vi "Parse And Send VISA Command String.vi"(8 "error in":errorcluster, 10 "command":string, 11 "VISA in":refnum<visa-resource-name>) -> (0 "error out":errorcluster, 2 "fetch data":T1[](array[typedef]), 3 "VISA out":refnum<visa-resource-name>)   [LabVIEW 2020]
uses:
  Raw VISA Read Data.ctl
  <vilib>/Instr/_visa.llb/VISA GPIB Control REN Mode.ctl
  <vilib>/Instr/_visa.llb/VISA Flush IO Buffer Mask.ctl
  Raw VISA Read Data.vi
  <vilib>/regexp/Match Regular Expression.xnode
  varilib/varilib.lvlib
panel:
  out "result string":string
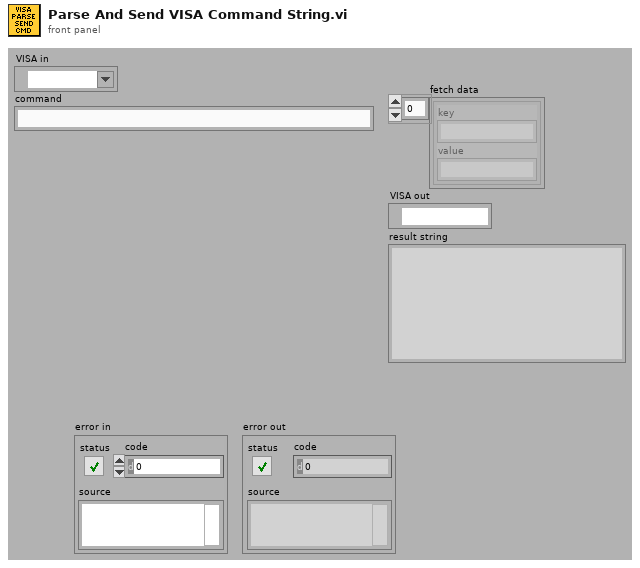
[diagram p1: front panel]
types:
  T1 = typedef "Raw VISA Read Data.ctl" = cluster{"key":string, "value":string}
  T2 = cluster{"submatch 2":string, "trimmed string":string}[]
  T3 = typedef "Raw VISA Read Data.vi" = cluster{"key":string, "value":string}
  T4 = typedef "VISA GPIB Control REN Mode.ctl" = u16
  T5 = typedef "VISA Flush IO Buffer Mask.ctl" = u16
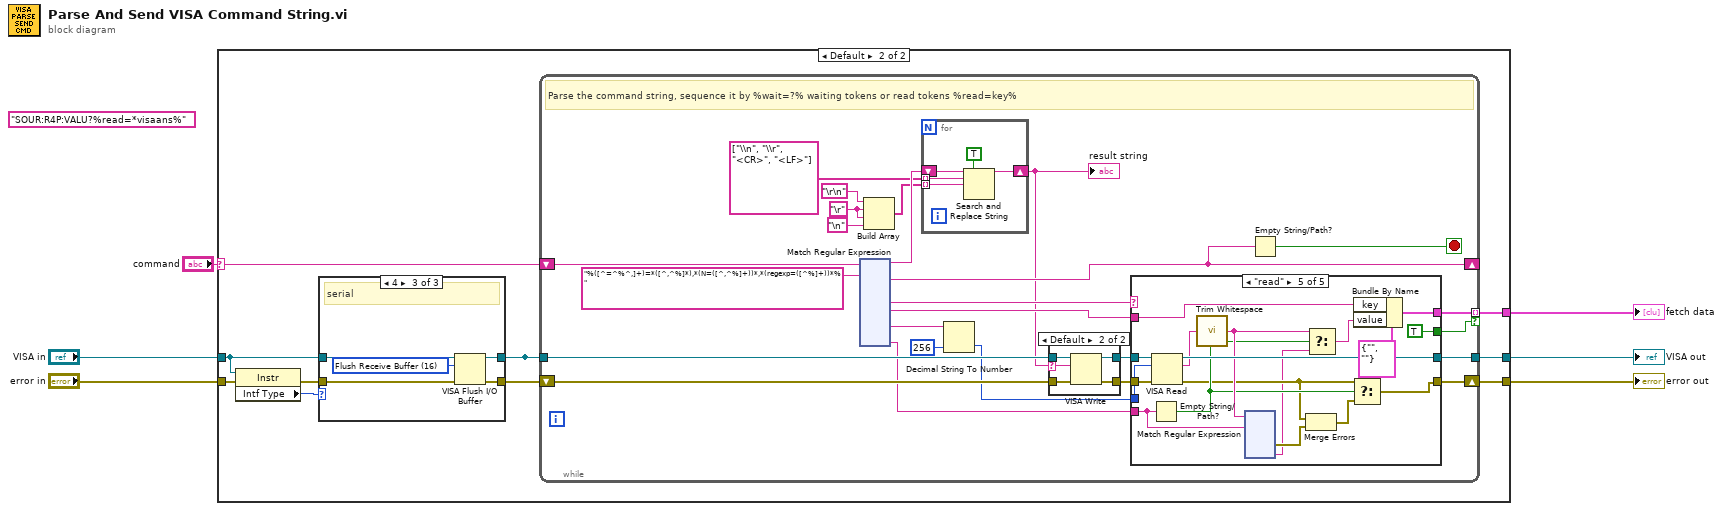
[diagram p0: block diagram]
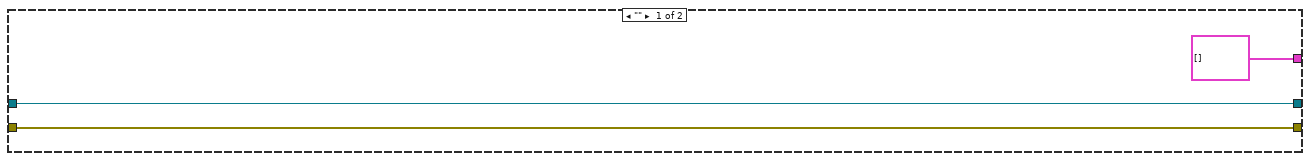
[diagram p2: hidden frame]
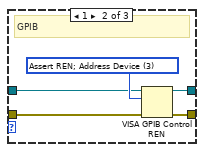
[diagram p4: hidden frame]
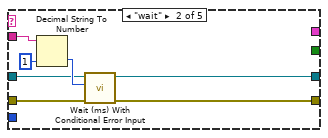
[diagram p7: hidden frame]
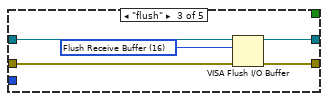
[diagram p8: hidden frame]
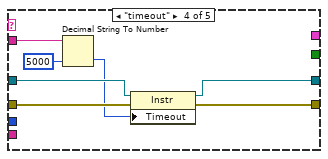
[diagram p9: hidden frame]
diagram:
  (unwired) "SOUR:R4P:VALU?%read=*visaans%"
  n1 = case shown="Default" "command" {
    selector: "command" -> [_ w17]
    tunnel: "error in" -> [w9 w12]
    tunnel: [w9 w18] -> w5
    tunnel: "VISA in" -> [w8 w13]
    tunnel: [w8 w15] -> w3
    tunnel: [T2 [] ("Array") w14] -> w4
    frame "" {
    }
    frame Default {
      n2 = property class="Instr"(reference=w13, error in=w12) -> (error out=w11:errorcluster, "Intf Type"=w10:u16)  [unwired: 1 out]
      n3 = case shown="4" w10 {
        tunnel: [w20 w25 w29] -> w16
        tunnel: [w19 w23 w28] -> w15
        tunnel: w13 -> [w19 w22 w27]
        tunnel: w11 -> [w20 w21 w30]
        frame 0, Default {
        }
        frame 1 {
          w24 = T4 3 items=["Deassert REN", "Assert REN", "Go To Local; Deassert REN ", "Assert REN; Address Device", "Local Lockout (Addressed Devices)", "Local Lockout (This Device)", "Go To Local"] ("Mode")
          # "GPIB"
          n4 = VISA GPIB Control REN(8:w21, 10:w24, 11:w22) -> (0:w25:errorcluster, 3:w23:refnum<visa-resource-name>)
        }
        frame 4 {
          w26 = T5 16 items=["Flush Receive Buffer"=16, "Write Transmit Buffer to Device"=32, "Flush Receive Buffer (No I/O)"=64, "Flush Transmit Buffer"=128] ("Mask")
          # "serial"
          n5 = VISA Flush I/O Buffer(VISA resource name=w27, mask (16)=w26, error in (no error)=w30) -> (VISA resource name out=w28:refnum<visa-resource-name>, error out=w29:errorcluster)
        }
      }
      n6 = while {
        shift-right: [w51] -> w18
        shift-left: w16 -> [w54]
        shift-right: [w49] -> _
        shift-left: w17 -> [w53]
        tunnel: w15 -> [w48]
        tunnel: [w46] -> _
        tunnel: [w43] -> w14 mode=indexing if=w42
        stop <- w50 stop-if-true
        w36 = "\r"
        # "Parse the command string, sequence it by %wait=?% waiting tokens or read tokens %read=key%"
        n7 = xnode "Match Regular Expression"("input string"=w53, "regular expression"="%([^=^%^,]+)=*([^,^%]*),*(N=([^,^%]+))*,*(regexp=([^%]+))*%") -> ("before match"=w41:string, "after match"=w49:string, "submatch 1"=w44:string, "submatch 2"=w45:string, "submatch 4"=w35:string, "submatch 6"=w32:string)  [unwired: 4 in, 5 out]
        n8 = Build Array("\r\n", w36, w36, "\n") -> (w39:string[])
        n9 = for {
          tunnel: string[] ["\\n", "\\r", "<CR>", "<LF>"] -> [w66] mode=indexing
          shift-right: [w64] -> w31
          shift-left: w41 -> [w67]
          tunnel: w39 -> [w63] mode=indexing
          n10 = Search and Replace String(replace all?=TRUE ("replace all? (F)"), input string=w67, search string=w66, replace string=w63) -> (result string=w64:string)  [unwired: 4 in, 3 out]
        }
        "result string" <- w31
        n11 = Decimal String To Number(string=w35, default (0L)=256 ("default (0 I32)")) -> (number=w33:i32)  [unwired: 1 in, 1 out]
        n12 = case shown="Default" w31 {
          selector: w31 -> [_ w58]
          tunnel: w54 -> [w56 w62]
          tunnel: [w56 w61] -> w52
          tunnel: w48 -> [w57 w60]
          tunnel: [w57 w59] -> w47
          frame "" {
          }
          frame Default {
            n13 = VISA Write(VISA resource name=w60, write buffer=w58, error in (no error)=w62) -> (VISA resource name out=w59:refnum<visa-resource-name>, error out=w61:errorcluster)  [unwired: 1 out]
          }
        }
        n14 = case shown="\"read\"" w44 {
          tunnel: w52 -> [w69 w75 w80 w87 w105]
          tunnel: [w69 w73 w77 w86 w90] -> w51
          tunnel: w47 -> [w68 w72 w78 w84 w104]
          tunnel: [w68 w72 w76 w85 w103] -> w46
          tunnel: w45 -> [_ w71 _ w83 w98]
          tunnel: [_ _ _ _ w101] -> w43
          tunnel: [_ _ _ _ TRUE] -> w42
          tunnel: w33 -> [_ _ _ _ w97]
          tunnel: w32 -> [_ _ _ _ w95]
          frame Default {
          }
          frame "wait" {
            n15 = Decimal String To Number(string=w71, default (0L)=1 ("default (0 I32)")) -> (number=w74:i32)  [unwired: 1 in, 1 out]
            n16 = call "Wait (ms) With Conditional Error Input.vi"("error in (no error)"=w75, "milliseconds to wait"=w74) -> ("error out"=w73:errorcluster)  [unwired: 8 in, 1 out]
          }
          frame "flush" {
            w79 = T5 16 items=["Flush Receive Buffer"=16, "Write Transmit Buffer to Device"=32, "Flush Receive Buffer (No I/O)"=64, "Flush Transmit Buffer"=128] ("Mask")
            n17 = VISA Flush I/O Buffer(VISA resource name=w78, mask (16)=w79, error in (no error)=w80) -> (VISA resource name out=w76:refnum<visa-resource-name>, error out=w77:errorcluster)
          }
          frame "timeout" {
            n18 = Decimal String To Number(string=w83, default (0L)=5000 ("default (0 I32)")) -> (number=w82:i32)  [unwired: 1 in, 1 out]
            n19 = property class="Instr"(reference=w84, error in=w87, "Timeout"=w82) -> (reference out=w85:refnum<visa-resource-name>, error out=w86:errorcluster)
          }
          frame "read" {
            n20 = Empty String/Path?(string/path=w95) -> (empty?=w94:bool)
            n21 = VISA Read(VISA resource name=w104, byte count=w97, error in (no error)=w105) -> (VISA resource name out=w103:refnum<visa-resource-name>, read buffer=w102:string, error out=w93:errorcluster)  [unwired: 1 out]
            n22 = call <vilib>:"Trim Whitespace.vi"("string"=w102) -> ("trimmed string"=w96:string)  [unwired: 1 in]
            n23 = xnode "Match Regular Expression"("input string"=w96, "regular expression"=w95) -> ("error out"=w92:errorcluster, "submatch 1"=w89:string)  [unwired: 4 in, 4 out]
            n24 = Merge Errors(w93, w92) -> (w91:errorcluster)
            n25 = Select(t=w96, s=w94, f=w89) -> (s? t:f=w88:string)
            n26 = Select(t=w93, s=w94, f=w91) -> (s? t:f=w90:errorcluster)
            n27 = Bundle By Name(cluster=T3 {"key"="", "value"=""} ("raw read data"), "key"=w98, "value"=w88) -> (w101:T3)
          }
        }
        n28 = Empty String/Path?(string/path=w49) -> (empty?=w50:bool)
      }
    }
  }
  "error out" <- w5
  "fetch data" <- w4
  "VISA out" <- w3
